vi "interactive trainer power check.vi"(11 "error in":errorcluster) -> (15 "error out":errorcluster)   [LabVIEW 2016]
doc: "this vi check the trainer power by reading the 5V rail via DAQ AI 3 and pops a dialog if the power isnt on.\n\nPaul K Dixon\nPhysics 350\nPaul K Dixon"
panel:
  # "interactive trainer power check"
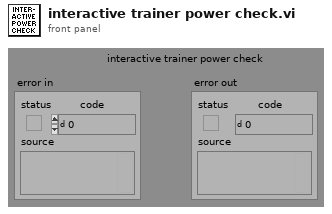
[diagram p1: front panel]
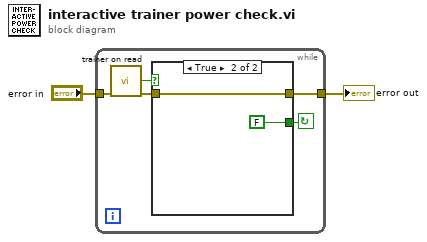
[diagram p0: block diagram]
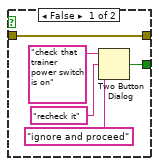
[diagram p2: hidden frame]
diagram:
  n1 = while {
    tunnel: [w3] -> w2
    tunnel: "error in" -> [w5]
    stop <- w6 continue-if-true
    n2 = call "trainer on read.vi"("error in (no error)"=w5) -> ("Trainer is on"=w7:bool, "error out"=w4:errorcluster)  [unwired: 13 out]
    n3 = case shown="True" w7 {
      tunnel: [w9 FALSE ("T button?")] -> w6
      tunnel: [w8 w13] -> w3
      tunnel: w4 -> [w8 w13]
      frame False {
        n4 = Two Button Dialog(message="check that trainer power switch is on", 1:"ignore and proceed" ("F button name (\"Cancel\")"), 2:"recheck it" ("T button name (\"OK\")")) -> (T button?=w9:bool)
      }
      frame True {
      }
    }
  }
  "error out" <- w2
